vi "PWM_Motor_IR.vi"(0 "Sensorwert":dbl, 1 "Start":bool, 2 "Sensorwert 2":dbl, 3 "Geschwindigkeit multiplikator":dbl(knob) scale=0.0..1.0) -> (6 "PWM Motor":dbl=0.3)   [LabVIEW 2016]
doc: "Geschwindigkeitsregelung anhand IR Sensor vorne\n05.04.17_Tloe"
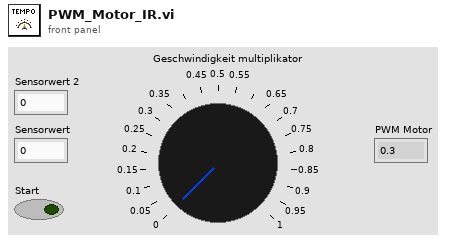
[diagram p1: front panel]
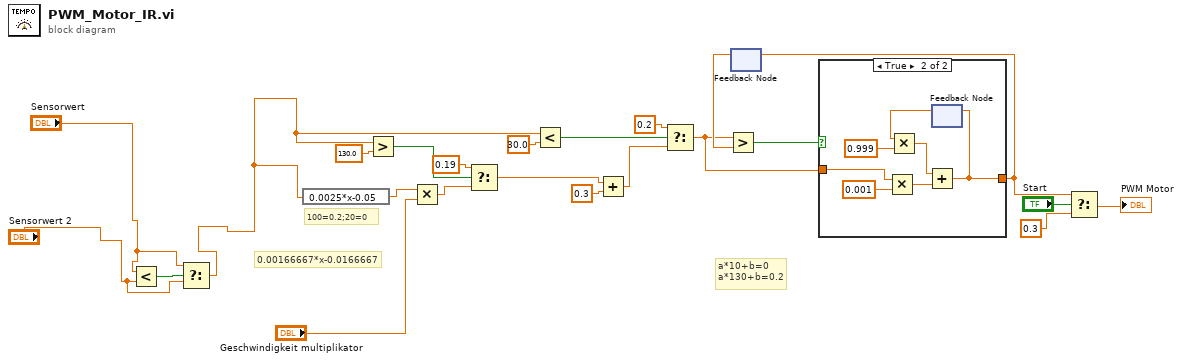
[diagram p0: block diagram]
diagram:
  # "100=0.2;20=0"
  # "0.00166667*x-0.0166667"
  # "a*10+b=0 \na*130+b=0.2"
  n1 = Less?(x="Sensorwert", y="Sensorwert 2") -> (x < y?=w11:bool)
  n2 = Select(t="Sensorwert", s=w11, f="Sensorwert 2") -> (s? t:f=w8:dbl)
  n3 = expression code="0.0025*x-0.05"(w8) -> (w3:dbl)
  n4 = Greater?(x=w8, y=130.0) -> (0:w22:bool)
  n5 = Multiply(x=w3, y="Geschwindigkeit multiplikator") -> (x*y=w2:dbl)
  n6 = Select(t=0.19, s=w22, f=w2) -> (s? t:f=w1:dbl)
  n7 = Less?(x=w8, y=30.0) -> (x < y?=w17:bool)
  n8 = Add(x=w1, y=0.3) -> (x+y=w18:dbl)
  n9 = Select(t=0.2, s=w17, f=w18) -> (s? t:f=w12:dbl)
  n10 = feedback #1() -> (w13:dbl)  [unwired: 1 in]
  n11 = Greater?(x=w12, y=w13) -> (0:w14:bool)
  n12 = case shown="True" w14 {
    tunnel: w12 -> [w24 w26]
    tunnel: [w24 w25] -> w6
    frame False {
    }
    frame True {
      n13 = Multiply(x=w26, y=0.001) -> (x*y=w28:dbl)
      n14 = feedback #2() -> (w31:dbl)  [unwired: 1 in]
      n15 = Multiply(x=w31, y=0.999) -> (x*y=w30:dbl)
      n16 = Add(x=w30, y=w28) -> (x+y=w25:dbl)
      n17 = feedback-in #2(w25) -> ()
    }
  }
  n18 = feedback-in #1(w6) -> ()
  n19 = Select(t=w6, s="Start", f=0.3) -> (s? t:f=→"PWM Motor":dbl)
